vi "dotNETChart Facade 1.vi"(0 "Data In":T11, 2 "Display State In":T2={"Chart Settings clstr"={"Enable Mouse Zoom (only works in 2D mode)"=TRUE, "Chart Wall Transparency Level"=37, "Chart Wall Colour"=0, "x axis label"="X axis title", "y axis label"="Y axis title", "Enable3D"=TRUE, "3D Settings"={"Inclination"=20, "LightStyle"=2, "Perspective"=4, "WallWidth"=5, "Rotation"=25}, "BackGradientStyle"=2, "SkinStyle"=1, "Chart Background Gradient Colour"=0, "Chart Border Colour"=0, "Palette"=12, "LegendStyle"=0, "ChartType"=[10, 13], "SeriesDataColour"=[]}} {"Chart Settings clstr"."ChartType" items=["Point", "FastPoint", "Bubble", "Line", "Spline", "StepLine", "FastLine", "Bar", "StackedBar", "StackedBar100", "Column", "StackedColumn", "StackedColumn100", "Area", "SplineArea", "StackedArea", "StackedArea100", "Pie", "Doughnut", "Stock", "Candlestick", "Range", "SplineRange", "RangeBar", "RangeColumn", "Radar", "Polar", "ErrorBar", "BoxPlot", "Renko", "ThreeLineBreak", "Kagi", "PointAndFigure", "Funnel", "Pyramid"]; "Chart Settings clstr"."LegendStyle" items=["Column", "Row", "Table"]; "Chart Settings clstr"."Palette" items=["None", "Bright", "Grayscale", "Excel", "Light", "Pastel", "EarthTones", "SemiTransparent", "Berry", "Chocolate", "Fire", "SeaGreen", "BrightPastel"]; "Chart Settings clstr"."SkinStyle" items=["None", "Emboss", "Raised", "Sunken", "FrameThin1", "FrameThin2", "FrameThin3", "FrameThin4", "FrameThin5", "FrameThin6", "FrameTitle1", "FrameTitle2", "FrameTitle3", "FrameTitle4", "FrameTitle5", "FrameTitle6", "FrameTitle7", "FrameTitle8"]; "Chart Settings clstr"."BackGradientStyle" items=["None", "LeftRight", "TopBottom", "Center", "DiagonalLeft", "DiagonalRight", "HorizontalCenter", "VerticalCenter"]; "Chart Settings clstr"."3D Settings"."LightStyle" items=["None", "Simplistic", "Realistic"]}, 3 "Container State":T10) -> (6 "Data Out":T11, 7 "Display State Out":T2={"Chart Settings clstr"={"Enable Mouse Zoom (only works in 2D mode)"=TRUE, "Chart Wall Transparency Level"=37, "Chart Wall Colour"=0, "x axis label"="X axis title", "y axis label"="Y axis title", "Enable3D"=TRUE, "3D Settings"={"Inclination"=20, "LightStyle"=2, "Perspective"=4, "WallWidth"=5, "Rotation"=25}, "BackGradientStyle"=2, "SkinStyle"=1, "Chart Background Gradient Colour"=0, "Chart Border Colour"=0, "Palette"=12, "LegendStyle"=0, "ChartType"=[10, 13], "SeriesDataColour"=[]}} {"Chart Settings clstr"."ChartType" items=["Point", "FastPoint", "Bubble", "Line", "Spline", "StepLine", "FastLine", "Bar", "StackedBar", "StackedBar100", "Column", "StackedColumn", "StackedColumn100", "Area", "SplineArea", "StackedArea", "StackedArea100", "Pie", "Doughnut", "Stock", "Candlestick", "Range", "SplineRange", "RangeBar", "RangeColumn", "Radar", "Polar", "ErrorBar", "BoxPlot", "Renko", "ThreeLineBreak", "Kagi", "PointAndFigure", "Funnel", "Pyramid"]; "Chart Settings clstr"."LegendStyle" items=["Column", "Row", "Table"]; "Chart Settings clstr"."Palette" items=["None", "Bright", "Grayscale", "Excel", "Light", "Pastel", "EarthTones", "SemiTransparent", "Berry", "Chocolate", "Fire", "SeaGreen", "BrightPastel"]; "Chart Settings clstr"."SkinStyle" items=["None", "Emboss", "Raised", "Sunken", "FrameThin1", "FrameThin2", "FrameThin3", "FrameThin4", "FrameThin5", "FrameThin6", "FrameTitle1", "FrameTitle2", "FrameTitle3", "FrameTitle4", "FrameTitle5", "FrameTitle6", "FrameTitle7", "FrameTitle8"]; "Chart Settings clstr"."BackGradientStyle" items=["None", "LeftRight", "TopBottom", "Center", "DiagonalLeft", "DiagonalRight", "HorizontalCenter", "VerticalCenter"]; "Chart Settings clstr"."3D Settings"."LightStyle" items=["None", "Simplistic", "Realistic"]}, 8 "Action":T1)   [LabVIEW 2013, in "dotNETChart XControl.xctl"]
uses:
  dotNETChart XControl.xctl
  dotNETChart Data 1.ctl
  <vilib>/_xctls/Container State.ctl
  dotNETChart State 1.ctl
  typedefs/ChartSettings cluster.ctl
  typedefs/3DSettings.ctl
  typedefs/BackGradientStyle.ctl
  typedefs/SkinStyle.ctl
  typedefs/Palette.ctl
  typedefs/LegendStyle.ctl
  typedefs/ChartType.ctl
  <vilib>/_xctls/Action.ctl
  <vilib>/_xctls/XControlSupport.lvlib
  System.Windows.Forms.DataVisualization
panel:
  in  "Microsoft Chart":refnum<k24>(container)
types:
  T1 = typedef "XControlSupport.lvlib/Action.ctl" = cluster{"Data Changed?":bool, "State Changed?":bool, "Action Name":string}
  T2 = typedef "dotNETChart XControl.xctl/dotNETChart State 1.ctl" = cluster{"Chart Settings clstr":T3}
  T3 = typedef "ChartSettings cluster.ctl" = cluster{"Enable Mouse Zoom (only works in 2D mode)":bool, "Chart Wall Transparency Level":i32, "Chart Wall Colour":u32, "x axis label":string, "y axis label":string, "Enable3D":bool, "3D Settings":T4, "BackGradientStyle":T5, "SkinStyle":T6, "Chart Background Gradient Colour":u32, "Chart Border Colour":u32, "Palette":T7, "LegendStyle":T8, "ChartType":T9[], "SeriesDataColour":u32[]}
  T4 = typedef "3DSettings.ctl" = cluster{"Inclination":i32, "LightStyle":i32, "Perspective":i32, "WallWidth":i32, "Rotation":i32}
  T5 = typedef "BackGradientStyle.ctl" = i32
  T6 = typedef "SkinStyle.ctl" = i32
  T7 = typedef "Palette.ctl" = i32
  T8 = typedef "LegendStyle.ctl" = i32
  T9 = typedef "ChartType.ctl" = i32
  T10 = typedef "XControlSupport.lvlib/Container State.ctl" = cluster{"Indicator?":bool, "Run Mode?":bool, " Refnum":refnum<vi>}
  T11 = typedef "dotNETChart XControl.xctl/dotNETChart Data 1.ctl" = dynamicdata
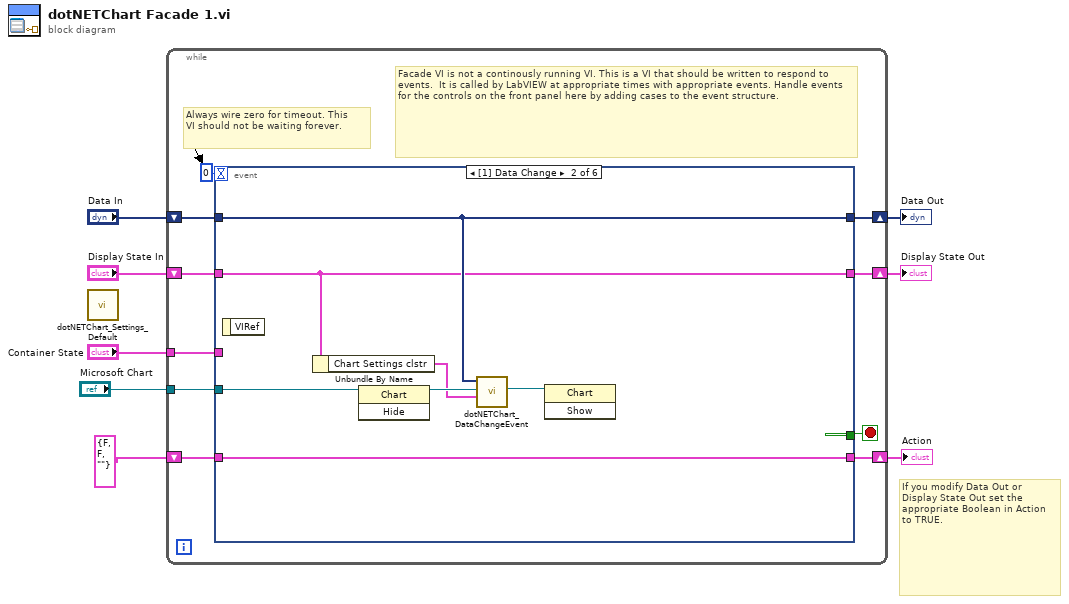
[diagram p0: block diagram]
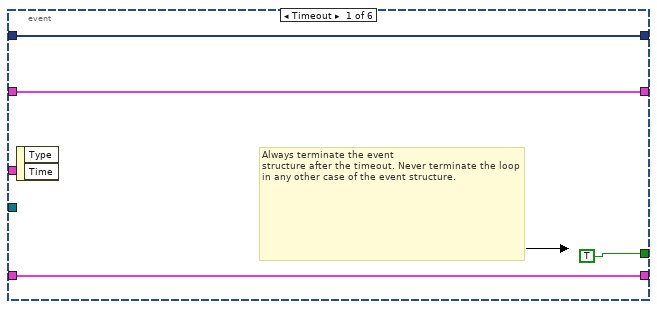
[diagram p2: hidden frame]
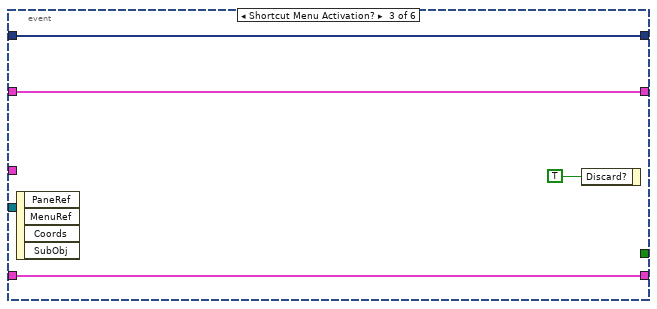
[diagram p3: hidden frame]
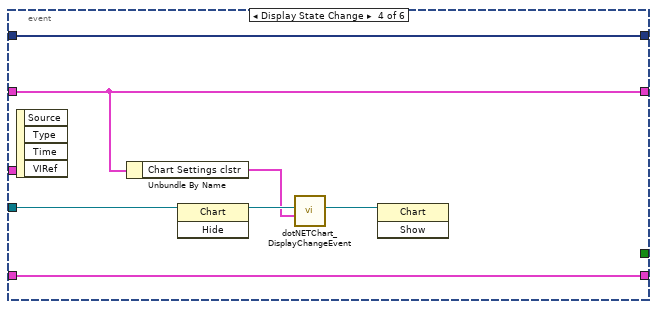
[diagram p4: hidden frame]
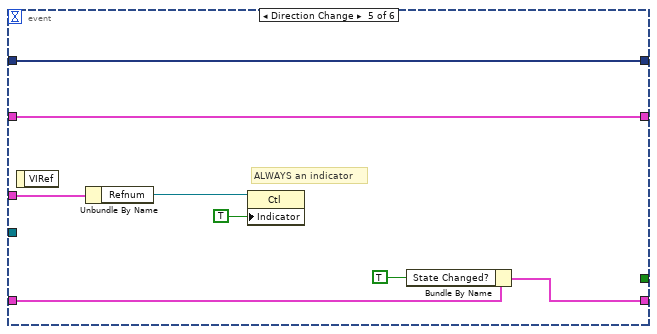
[diagram p5: hidden frame]
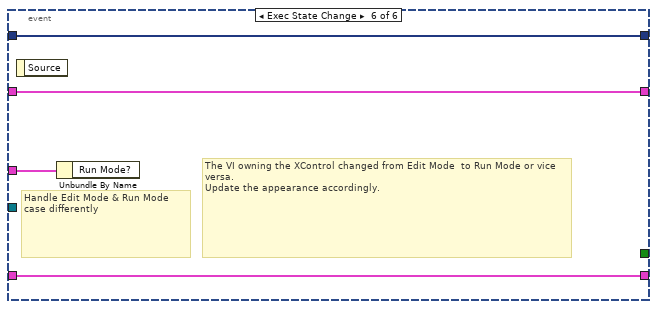
[diagram p6: hidden frame]
diagram:
  # "If you modify Data Out or\nDisplay State Out set the\nappropriate Boolean in Action\nto TRUE."
  n1 = call "dotNETChart_Settings_Default.vi"() -> ()  [unwired: 11 in, 1 out]
  n2 = while {
    shift-right: [w17] -> w5
    shift-left: "Display State In" -> [w18]
    tunnel: "Container State" -> [w14]
    shift-right: [w12] -> w8
    shift-left: "Data In" -> [w13]
    shift-right: [w10] -> w4
    shift-left: T1 {"Data Changed?"=FALSE, "State Changed?"=FALSE, "Action Name"=""} ("Action") -> [w11]
    tunnel: "Microsoft Chart" -> [w9]
    stop <- w16 stop-if-true
    # "Facade VI is not a continously running VI. This is a VI that should be written to respond to events.  It is called by LabVIEW at appropriate times with appropriate events. Handle events for the controls on the front panel here by adding cases to the event structure."
    # "Always wire zero for timeout. This\nVI should not be waiting forever."
    n3 = event shown="[1] Data Change" {
      selector: _ -> [_ _ _ _ _ _]
      dyn-events: _ -> [_ _ _ _ _ _]
      timeout: 0 -> [_ _ _ _ _ _]
      tunnel: w18 -> [w20 w24 w32 w37 w41 w51]
      tunnel: [w20 w24 w32 w37 w41 w51] -> w17
      tunnel: [TRUE _ _ _ _ _] -> w16
      tunnel: w14 -> [_ _ _ _ w48 w52]
      tunnel: w13 -> [w19 w27 w33 w40 w47 w50]
      tunnel: [w19 w27 w33 w40 w47 w50] -> w12
      tunnel: [w21 w29 w31 w39 w45 w49] -> w10
      tunnel: w11 -> [w21 w29 w31 w39 w44 w49]
      tunnel: w9 -> [_ w28 _ w38 _ _]
      event Timeout {
        # "Always terminate the event\nstructure after the timeout. Never terminate the loop in any other case of the event structure."
        n4 = event-data() -> ()  [unwired: 1 in, 2 out]
      }
      event Data Change {
        n5 = event-data() -> ()  [unwired: 1 in, 1 out]
        n6 = Unbundle By Name(w24) -> ("Chart Settings clstr"=w23:T3)
        n7 = invoke class="Chart" method="Hide"(reference=w28) -> (reference out=w26:refnum<k24>)  [unwired: 2 in, 2 out]
        n8 = call "dotNETChart_DataChangeEvent.vi"("Chart Settings clstr"=w23, "Microsoft Chart"=w26, "chart data"=w27) -> ("reference out"=w25:refnum<k24>)  [unwired: 7 in, 1 out]
        n9 = invoke class="Chart" method="Show"(reference=w25) -> ()  [unwired: 2 in, 3 out]
      }
      event Shortcut Menu Activation? {
        n10 = event-data() -> ()  [unwired: 1 in, 4 out]
        n11 = event-data("Discard?"=TRUE) -> ()  [unwired: 1 in, 1 out]
      }
      event Display State Change {
        n12 = event-data() -> ()  [unwired: 1 in, 4 out]
        n13 = Unbundle By Name(w37) -> ("Chart Settings clstr"=w34:T3)
        n14 = invoke class="Chart" method="Hide"(reference=w38) -> (reference out=w36:refnum<k24>)  [unwired: 2 in, 2 out]
        n15 = call "dotNETChart_DisplayChangeEvent.vi"("Chart Settings clstr"=w34, "Microsoft Chart"=w36) -> ("reference out"=w35:refnum<k24>)  [unwired: 8 in, 1 out]
        n16 = invoke class="Chart" method="Show"(reference=w35) -> ()  [unwired: 2 in, 3 out]
      }
      event Direction Change {
        # "ALWAYS an indicator"
        n17 = event-data() -> ()  [unwired: 1 in, 1 out]
        n18 = Unbundle By Name(w48) -> ("Refnum"=w46:refnum<vi>)
        n19 = property class="Ctl"(reference=w46, "Indicator"=TRUE) -> ()  [unwired: 1 in, 2 out]
        n20 = Bundle By Name(cluster=w44, "State Changed?"=TRUE) -> (w45:T1)
      }
      event Exec State Change {
        # "The VI owning the XControl changed from Edit Mode  to Run Mode or vice versa.\nUpdate the appearance accordingly."
        # "Handle Edit Mode & Run Mode\ncase differently"
        n21 = event-data() -> ()  [unwired: 1 in, 1 out]
        n22 = Unbundle By Name(w52) -> ()  [unwired: 1 out]
      }
    }
  }
  "Display State Out" <- w5
  "Data Out" <- w8
  "Action" <- w4
